vi "Example.vi"() -> ()   [LabVIEW 2017]
doc: "Code originally found in this LAVA thread.\n\nhttps://lavag.org/topic/19236-turn-your-front-panel-into-an-interactive-html5-site/\n\nModified by Hooovahh"
uses:
  FP Publisher/Common/Enum - Config Option.ctl
  FP Publisher/Web Front Panel_class/Controls/High Level Config Settings.ctl
  <vilib>/Platform/browser.llb/Open URL in Default Browser (path).vi
  <vilib>/Analysis/3filter.llb/FIR Filter (DBL).vi
  FP Publisher/Front Panel Publisher.lvlib
  <vilib>/Analysis/NI_AALBase.lvlib
  FP Publisher/Web Front Panel_class/Web Front Panel.lvclass
panel:
  in  "Cluster Outer":T1={"Cluster Inner"={"Test Button"=FALSE, "Test String Inner"="123"}, "Test String Outer"="456"}
  in  "Close All":bool
  in  "Open All":bool
  out "String Indicator 2":string
  in  "Tree Indicator":string(tree)
  in  "Hide":bool
  in  "Show":bool
  in  "Update":bool
  out "Status":bool
  out "Picture Ring 2":u16(ring)
  in  "String Control":string="abcd"
  out "String Indicator":string="abcd"
  out "Picture Ring 1":u16(ring)
  out "Progress":dbl(slide)=3.1645569620253164 scale=0.0..10.0
  out "Path Indicator":path=path "C:/temp/log.txt"
  in  "Averaging":enum16{"5pt", "11pt", "33pt"}(ring)
  out "<5":bool
  in  "Button":bool
  in  "Stop":bool
  out "XY Graph":cluster{i32[], "Filtered X":dbl[]}[](graph)
  in  "Append":bool
  in  "Numeric":dbl
  out "Label":string="Hardware ABCD"
  # "Floating Text"
  # "Other"
  # "Sizes"
  # "Bolded"
  # "By default all of these controls only send their value, or their value and position with each request except for the Path Indicator and Tree"
  # "Indicator which is represented as an image.  These two images sends over 170KB of data with each request, with all other controls combined"
  # "only around 800 bytes.  This is why sending controls as images should only be used when other options don't work."
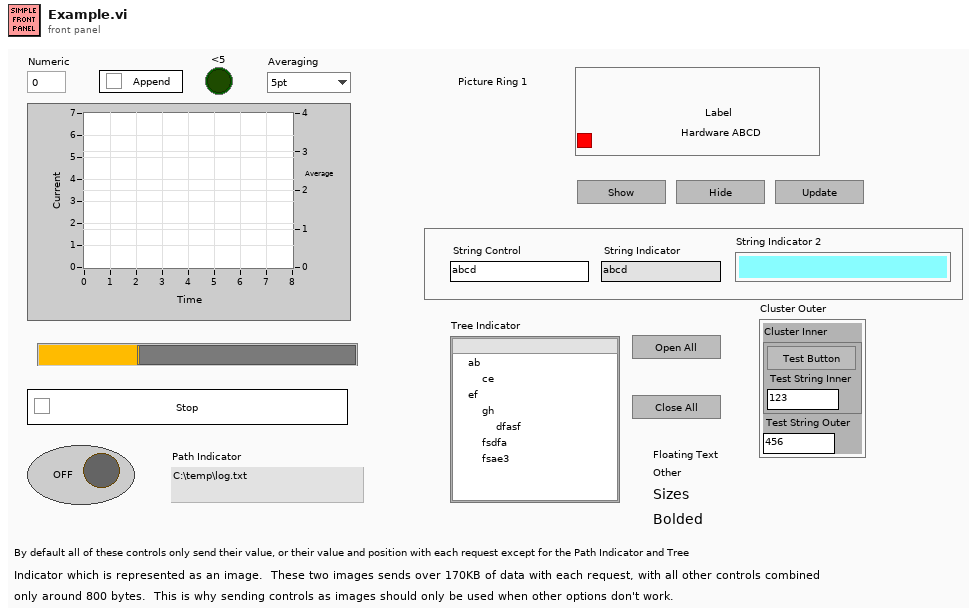
[diagram p1: front panel]
types:
  T1 = cluster{"Cluster Inner":cluster{"Test Button":bool, "Test String Inner":string}, "Test String Outer":string}
  T2 = typedef "Front Panel Publisher.lvlib/Web Front Panel.lvclass/High Level Config Settings.ctl" = cluster{"Default Refresh Rate (ms)":i32, "Show Border":bool, "Periodic Decoration Data":bool, "Synchronous Requests":bool, "Reduce Sent Data":bool, "Recommended Control Settings":bool}
  T3 = typedef "Front Panel Publisher.lvlib/Enum - Config Option.ctl" = enum16{"Show Config Dialog", "Don't Show Config Dialog", "Load Config File then Show Dialog", "Load Config File No Dialog"}
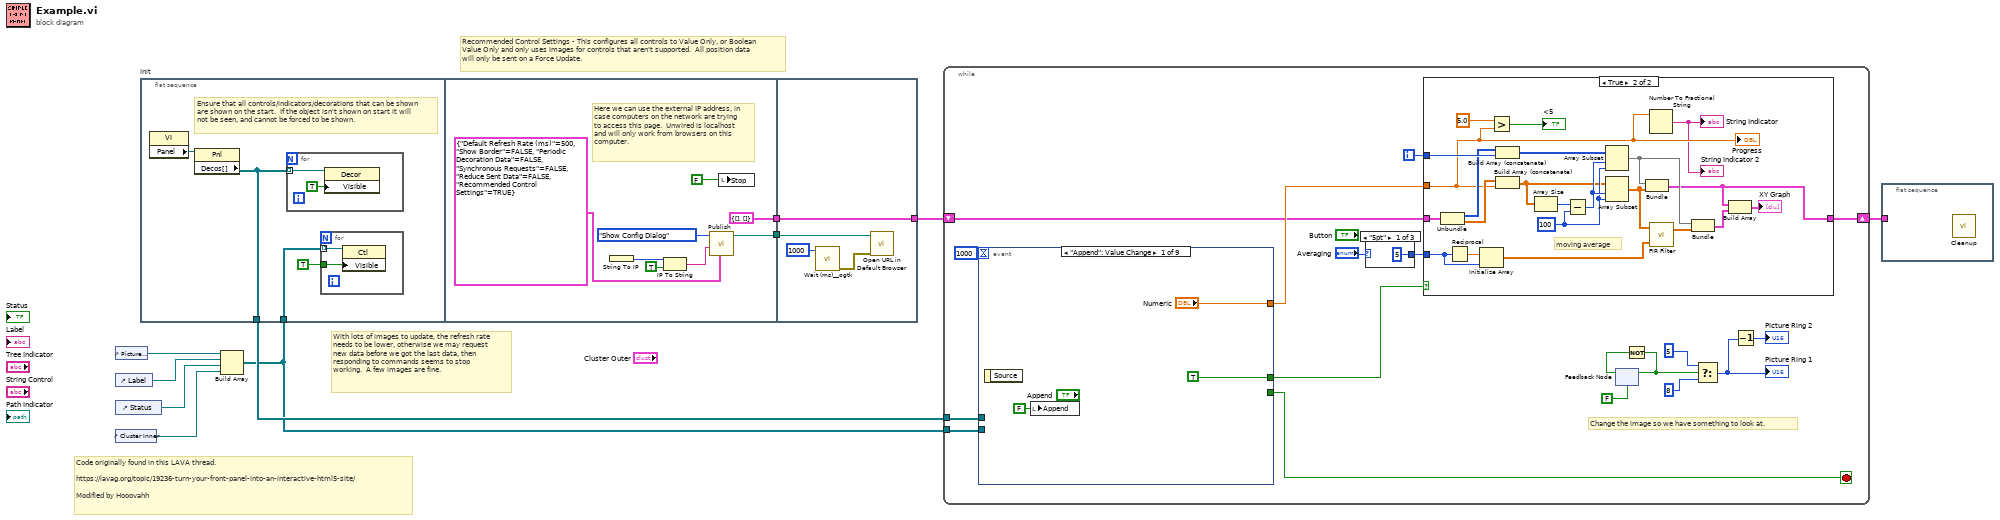
[diagram p0: block diagram]
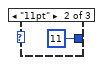
[diagram p2: hidden frame]
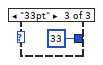
[diagram p3: hidden frame]
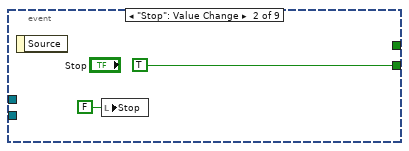
[diagram p5: hidden frame]
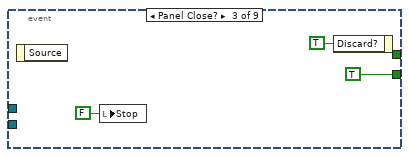
[diagram p6: hidden frame]
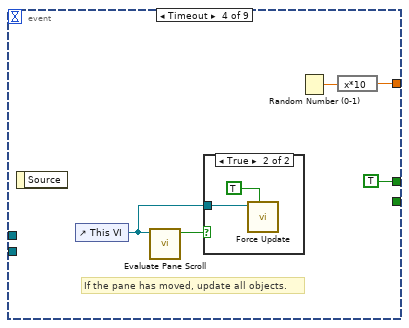
[diagram p7: hidden frame]
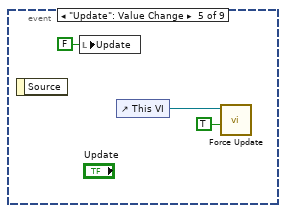
[diagram p9: hidden frame]
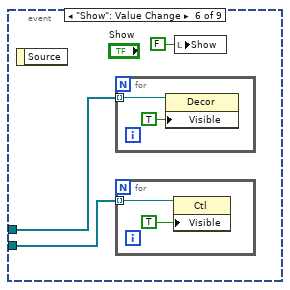
[diagram p10: hidden frame]
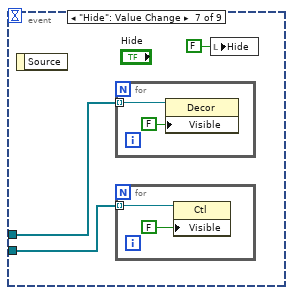
[diagram p11: hidden frame]
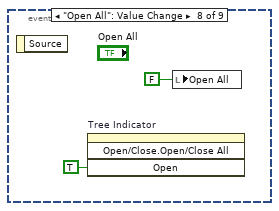
[diagram p12: hidden frame]
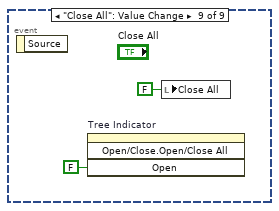
[diagram p13: hidden frame]
diagram:
  # "Recommended Control Settings - This configures all controls to Value Only, or Boolean Value Only and only uses Images for controls that aren't supported.  All position data will only be sent on a Force Update."
  # "Code originally found in this LAVA thread.\n\nhttps://lavag.org/topic/19236-turn-your-front-panel-into-an-interactive-html5-site/\n\nModified by Hooovahh"
  # "With lots of images to update, the refresh rate needs to be lower, otherwise we may request new data before we got the last data, then responding to commands seems to stop working.  A few images are fine."
  n1 = control-ref of="Picture Ring 2"() -> (w7:refnum<vi>)
  n2 = control-ref of="Label"() -> (w6:refnum<vi>)
  n3 = control-ref of="Status"() -> (w8:refnum<vi>)
  n4 = control-ref of="Cluster Inner"() -> (w3:refnum<vi>)
  n5 = flat-sequence "Init" {
    tunnel: w1 -> [w14]
    tunnel: [w11] -> w2
    tunnel: [cluster{i32[], dbl[]} {[], []} ("XY Graph")] -> w5
    tunnel: [w22] -> w4
    tunnel: [w30] -> w10
    tunnel: w5 -> [w30]
    tunnel: w4 -> [w29]
    frame #0 {
      # "Ensure that all controls/indicators/decorations that can be shown are shown on the start.  If the object isn't shown on start it will not be seen, and cannot be forced to be shown."
      n6 = property class="VI"() -> ("Panel"=w12:refnum<vi>)  [unwired: 2 in, 2 out]
      n7 = property class="Pnl"(reference=w12) -> ("Decos[]"=w11:refnum<vi>[])  [unwired: 1 in, 2 out]
      n8 = for {
        tunnel: w11 -> [w15] mode=indexing
        n9 = property class="Decor"(reference=w15, "Visible"=TRUE) -> ()  [unwired: 1 in, 2 out]
      }
      n10 = for {
        tunnel: w14 -> [w17] mode=indexing
        tunnel: TRUE -> [w18]
        n11 = property class="Ctl"(reference=w17, "Visible"=w18) -> ()  [unwired: 1 in, 2 out]
      }
    }
    frame #1 {
      # "Here we can use the external IP address, in case computers on the network are trying to access this page.  Unwired is localhost and will only work from browsers on this computer."
      n12 = String To IP() -> (0:w23:u32)  [unwired: 1 in]
      n13 = IP To String(1:TRUE ("dot notation? (F)"), 2:w23) -> (0:w19:string)
      n14 = call "Publish.vi"("High Level Config Settings"=T2 {"Default Refresh Rate (ms)"=500, "Show Border"=FALSE, "Periodic Decoration Data"=FALSE, "Synchronous Requests"=FALSE, "Reduce Sent Data"=FALSE, "Recommended Control Settings"=TRUE}, "Host Connection"=w19, "Config Option"=Enum_-_Config_Option."Show Config Dialog") -> ("Created HTML"=w22:path)  [unwired: 6 in, 2 out]
      n15 = local write "Stop"(FALSE ("Stop")) -> ()
    }
    frame #2 {
      n16 = call <userlib>:"Wait (ms)__ogtk.vi"("milliseconds to wait"=u32 1000) -> ("error out"=w28:errorcluster)  [unwired: 9 in, 1 out]
      n17 = call-poly <vilib>:"Open URL in Default Browser.vi"("error in (no error)"=w28, "path"=w29) -> ()  [unwired: 4 in, 2 out]
    }
  }
  n18 = Build Array(w7, w6, w8, w3) -> (w1:refnum<vi>[])
  n19 = while {
    shift-right: [w43] -> w9
    shift-left: w10 -> [w42]
    tunnel: w2 -> [w32]
    tunnel: w1 -> [w31]
    i -> [w45]
    stop <- w48 stop-if-true
    # "Change the image so we have something to look at."
    n20 = event shown="[0] \"Append\": Value Change" {
      selector: _ -> [_ _ _ _ _ _ _ _ _]
      dyn-events: _ -> [_ _ _ _ _ _ _ _ _]
      timeout: 1000 -> [_ _ _ _ _ _ _ _ _]
      tunnel: [_ TRUE TRUE _ _ _ _ _ _] -> w48
      tunnel: ["Numeric" _ _ w86 _ _ _ _ _] -> w44
      tunnel: [TRUE _ _ TRUE _ _ _ _ _] -> w46
      tunnel: w32 -> [_ _ _ _ _ w94 w101 _ _]
      tunnel: w31 -> [_ _ _ _ _ w93 w100 _ _]
      event "Append": Value Change {
        n21 = event-data() -> ()  [unwired: 1 in, 1 out]
        n22 = local write "Append"(FALSE ("Add")) -> ()
      }
      event "Stop": Value Change {
        n23 = event-data() -> ()  [unwired: 1 in, 1 out]
        n24 = local write "Stop"(FALSE ("Stop")) -> ()
      }
      event Panel Close? {
        n25 = event-data() -> ()  [unwired: 1 in, 1 out]
        n26 = local write "Stop"(FALSE ("Stop")) -> ()
        n27 = event-data("Discard?"=TRUE) -> ()  [unwired: 1 in, 1 out]
      }
      event Timeout {
        # "If the pane has moved, update all objects."
        n28 = event-data() -> ()  [unwired: 1 in, 1 out]
        n29 = control-ref of="This VI"() -> (w83:refnum<vi>)
        n30 = call "Evaluate Pane Scroll.vi"("VI Reference"=w83) -> ("Pane Scrolled"=w84:bool)  [unwired: 9 in, 1 out]
        n31 = case shown="True" w84 {
          tunnel: w83 -> [_ w88]
          frame False {
          }
          frame True {
            n32 = call "Force Update.vi"("Update Origin"=TRUE, "VI Refnum"=w88) -> ()  [unwired: 10 in]
          }
        }
        n33 = Random Number (0-1)() -> (number: 0 to 1=w87:dbl)
        n34 = expression code="x*10"(w87) -> (w86:dbl)
      }
      event "Update": Value Change {
        n35 = event-data() -> ()  [unwired: 1 in, 1 out]
        n36 = local write "Update"(FALSE ("Update")) -> ()
        n37 = control-ref of="This VI"() -> (w91:refnum<vi>)
        n38 = call "Force Update.vi"("All Controls and Decorations"=TRUE, "VI Refnum"=w91) -> ()  [unwired: 10 in]
      }
      event "Show": Value Change {
        n39 = event-data() -> ()  [unwired: 1 in, 1 out]
        n40 = for {
          tunnel: w94 -> [w99] mode=indexing
          n41 = property class="Decor"(reference=w99, "Visible"=TRUE) -> ()  [unwired: 1 in, 2 out]
        }
        n42 = for {
          tunnel: w93 -> [w97] mode=indexing
          n43 = property class="Ctl"(reference=w97, "Visible"=TRUE) -> ()  [unwired: 1 in, 2 out]
        }
        n44 = local write "Show"(FALSE ("Show")) -> ()
      }
      event "Hide": Value Change {
        n45 = event-data() -> ()  [unwired: 1 in, 1 out]
        n46 = for {
          tunnel: w101 -> [w106] mode=indexing
          n47 = property class="Decor"(reference=w106, "Visible"=FALSE) -> ()  [unwired: 1 in, 2 out]
        }
        n48 = for {
          tunnel: w100 -> [w104] mode=indexing
          n49 = property class="Ctl"(reference=w104, "Visible"=FALSE) -> ()  [unwired: 1 in, 2 out]
        }
        n50 = local write "Hide"(FALSE ("Hide")) -> ()
      }
      event "Open All": Value Change {
        n51 = event-data() -> ()  [unwired: 1 in, 1 out]
        n52 = invoke on="Tree Indicator" class="Tree (strict)" method="Open/Close.Open/Close All"("Open"=TRUE ("Open?")) -> ()  [unwired: 3 in, 4 out]
        n53 = local write "Open All"(FALSE ("Expand All")) -> ()
      }
      event "Close All": Value Change {
        n54 = event-data() -> ()  [unwired: 1 in, 1 out]
        n55 = invoke on="Tree Indicator" class="Tree (strict)" method="Open/Close.Open/Close All"("Open"=FALSE ("Open?")) -> ()  [unwired: 3 in, 4 out]
        n56 = local write "Close All"(FALSE ("Close All")) -> ()
      }
    }
    n57 = case shown="\"5pt\"" "Averaging" {
      tunnel: [5 11 33] -> w41
      frame "5pt" {
      }
      frame "11pt" {
      }
      frame "33pt" {
      }
    }
    n58 = case shown="True" w46 {
      tunnel: w45 -> [_ w74]
      tunnel: w44 -> [_ w54]
      tunnel: [w52 w61] -> w43
      tunnel: w42 -> [w52 w73]
      tunnel: w41 -> [_ w56]
      frame False {
      }
      frame True {
        w68 = 100 ("length")
        # "moving average"
        n59 = Unbundle(w73) -> (w71:i32[], w67:dbl[])
        n60 = Reciprocal(x=w56) -> (1/x=w58:dbl)
        n61 = Initialize Array(w58, w56) -> (w57:dbl[])
        n62 = Greater?(x=5.0, y=w54) -> (0:→"<5":bool)
        n63 = Build Array (concatenate)(w71, w74) -> (w72:i32[])
        n64 = Build Array (concatenate)(w67, w54) -> (w66:dbl[])
        n65 = Array Size(array=w66) -> (size(s)=w70:i32)
        n66 = Subtract(x=w70, y=w68) -> (x-y=w69:i32)
        n67 = Array Subset(array=w72, index=w69, length=w68) -> (w63:i32[])
        n68 = Array Subset(array=w66, index=w69, length=w68) -> (w60:dbl[])
        n69 = Bundle(w63, w60) -> (w61:cluster{i32[], dbl[]})  [unwired: 1 in]
        n70 = Number To Fractional String(number=w54) -> (F-format string=→"String Indicator" →"String Indicator 2":string)  [unwired: 3 in]
        n71 = call-poly <vilib>:"FIR Filter.vi"("FIR Coefficients"=w57, "X"=w60) -> ("Filtered X"=w59:dbl[])  [unwired: 2 in, 1 out]
        n72 = Bundle(w63, "Filtered X"=w59) -> (w62:cluster{i32[], "Filtered X":dbl[]})  [unwired: 1 in]
        n73 = Build Array(w61, w62) -> (→"XY Graph":cluster{i32[], "Filtered X":dbl[]}[])
        "Progress" <- w54
      }
    }
    n74 = feedback #1(FALSE) -> (w38:bool)
    n75 = Not(x=w38) -> (.not. x?=w35:bool)
    n76 = feedback-in #1(w35) -> ()
    n77 = Select(t=u32 5 ("Number of Rows"), s=w35, f=u32 8 ("Number of Rows")) -> (s? t:f=w34:u32)
    "Picture Ring 1" <- w34
    n78 = Decrement(x=w34) -> (x-1=→"Picture Ring 2":u32)
  }
  n79 = flat-sequence {
    tunnel: w9 -> [_]
    frame #0 {
      n80 = call "Cleanup.vi"() -> ()  [unwired: 11 in, 1 out]
    }
  }
